vi "Write Other Refs.vi"(8 "error in (no error)":errorcluster, 10 "Refs":T1, 11 "teststand-api in":refnum<class "teststand-api.lvclass">) -> (0 "error out":errorcluster, 3 "teststand-api out":refnum<class "teststand-api.lvclass">)   [LabVIEW 2014, in "teststand-api.lvlib" / "teststand-api.lvclass"]
uses:
  teststand-api.lvclass
  Other Refs Argument--cluster.ctl
  Process Model--cluster.ctl
  Model Run Mode--enum.ctl
  teststand-api.lvclass/teststand-api.ctl
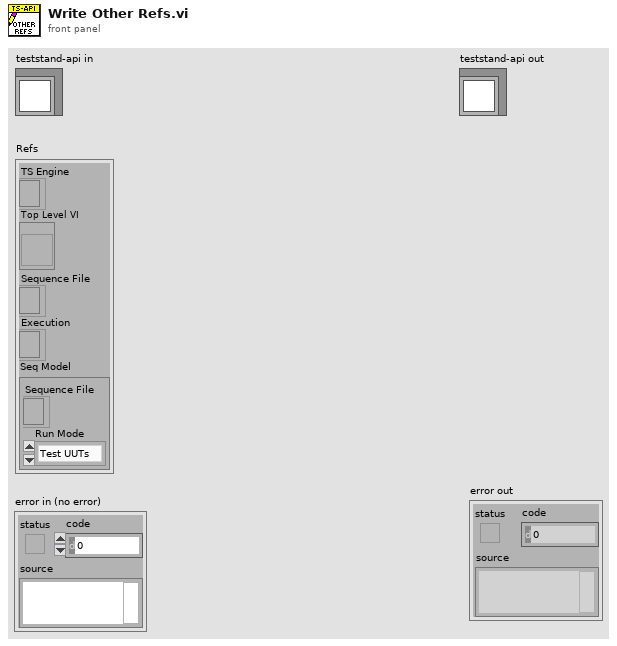
[diagram p1: front panel]
types:
  T1 = typedef "teststand-api.lvlib/teststand-api.lvclass/Other Refs Argument--cluster.ctl" = cluster{"TS Engine":refnum<k7>, "Top Level VI ":refnum<vi>, "Sequence File":refnum<k7>, "Execution":refnum<k7>, "Seq Model":T2}
  T2 = typedef "teststand-api.lvlib/teststand-api.lvclass/Process Model--cluster.ctl" = cluster{"Sequence File":refnum<k7>, "Run Mode":T3}
  T3 = typedef "teststand-api.lvlib/teststand-api.lvclass/Model Run Mode--enum.ctl" = enum16{"Test UUTs", "Single Pass"}
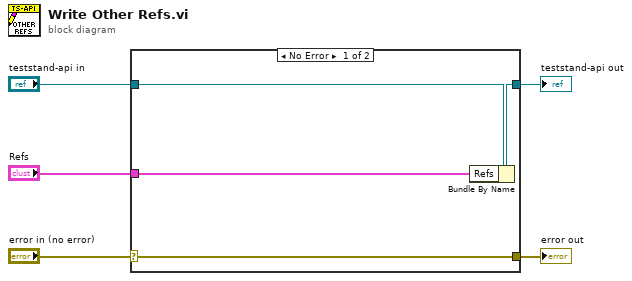
[diagram p0: block diagram]
diagram:
  n1 = case shown="No Error" "error in (no error)" {
    selector: "error in (no error)" -> [w9 w10]
    tunnel: [w9 w10] -> w4
    tunnel: [w7 w11] -> w2
    tunnel: "teststand-api in" -> [w8 w11]
    tunnel: "Refs" -> [w6 _]
    frame No Error {
      n2 = Bundle By Name(cluster=w8, "Refs"=w6) -> (w7:refnum<class "teststand-api.lvclass">)
    }
    frame Error {
    }
  }
  "error out" <- w4
  "teststand-api out" <- w2
